vi "AutoTurnOneSide.vi"() -> ()   [LabVIEW 2014]
uses:
  Robot Global Data.vi
panel:
  in  "Desired Right Inches":dbl
  in  "Desired Left Inches":dbl
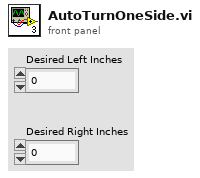
[diagram p1: front panel]
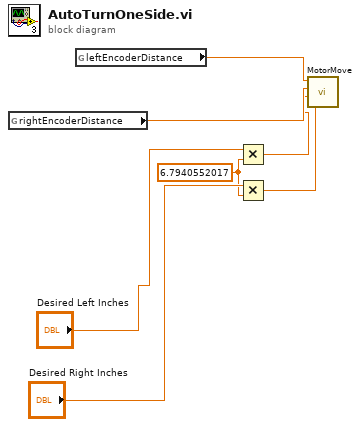
[diagram p0: block diagram]
diagram:
  w5 = 6.7940552017 ("y")
  n1 = global read "Robot Global Data.vi" "rightEncoderDistance"() -> (w3:dbl)
  n2 = global read "Robot Global Data.vi" "leftEncoderDistance"() -> (w4:dbl)
  n3 = Multiply(x="Desired Left Inches", y=w5) -> (x*y=w2:dbl)
  n4 = Multiply(x="Desired Right Inches", y=w5) -> (x*y=w1:dbl)
  n5 = call "MotorMove.vi"("Left Enc. Distance"=w4, "Right Enc. Distance"=w3, "Left Desired"=w2, "Right Desired"=w1) -> ()  [unwired: 6 in]
